vi "solar_voy Valid Refnum.vi"(1 "Voyager Refnum":T1) -> (0 "Invalid Refnum?":bool)   [LabVIEW 2018]
doc: "This checks if the Voyager reference is invalid."
uses:
  solar_voy_def/solar_voy_def_ctl PACKET_ID.ctl
  solar_voy_ctl Voyager.ctl
  type/solar_type Item Type.ctl
  solar_voy_def/solar_voy_def_ctl ITEM TYPE.ctl
  solar_voy_def/solar_voy_def_ctl ITEM.ctl
  solar_voy_def/solar_voy_def_ctl PACKET.ctl
  solar_voy_ctl TCP.ctl
  solar_voy_def/solar_voy_def_ctl HDR.ctl
  solar_voy_ctl Port Setup.ctl
  solar_voy_ctl Voyager Refnum.ctl
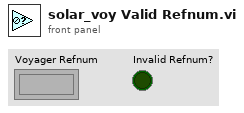
[diagram p1: front panel]
types:
  T1 = typedef "solar_voy_ctl Voyager Refnum.ctl" = refnum<k1>
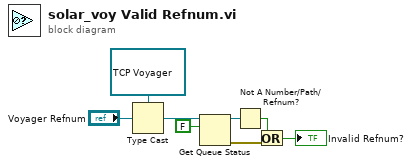
[diagram p0: block diagram]
diagram:
  n1 = Type Cast(type=refnum<queue> refnum ("Voyager SEQ"), x="Voyager Refnum") -> (*(type *) &x=w2:refnum<queue>)
  n2 = Get Queue Status(queue=w2, return elements? (F)=FALSE) -> (queue out=w3:refnum<queue>, error out=w4:errorcluster)  [unwired: 1 in, 6 out]
  n3 = Not A Number/Path/Refnum?(number/path/refnum=w3) -> (NaN/Path/Refnum?=w5:bool)
  n4 = Or(x=w5, y=w4) -> (x .or. y?=→"Invalid Refnum?":bool)
